vi "multi_channel_DO.vi"(5 "data":u8[][](array[numeric]), 6 "sample num":i32=1000, 7 "sample rate":dbl=1000.0 format="%0.2f", 8 "edge":i32(ring)=10280 items=["上升"=10280, "下降"=10171], 9 "trigger channel":tag, 10 "Trigger Type":enum32{"No Trigger", "Digital Start"}(ring), 11 "channels":tag) -> ()   [LabVIEW 2019]
uses:
  <vilib>/DAQmx/write.llb/DAQmx Write (Digital Wfm 1Chan NSamp).vi
  <vilib>/DAQmx/create/channels.llb/DAQmx Create Channel (DO-Digital Output).vi
  <vilib>/DAQmx/configure/timing.llb/DAQmx Timing (Sample Clock).vi
  <vilib>/DAQmx/configure/trigger.llb/DAQmx Start Trigger (Digital Edge).vi
  <vilib>/Waveform/DWDTOps.llb/DWDT Uncompress Digital.vi
  <vilib>/DAQmx/miscellaneous.llb/DAQmx Fill In Error Info.vi
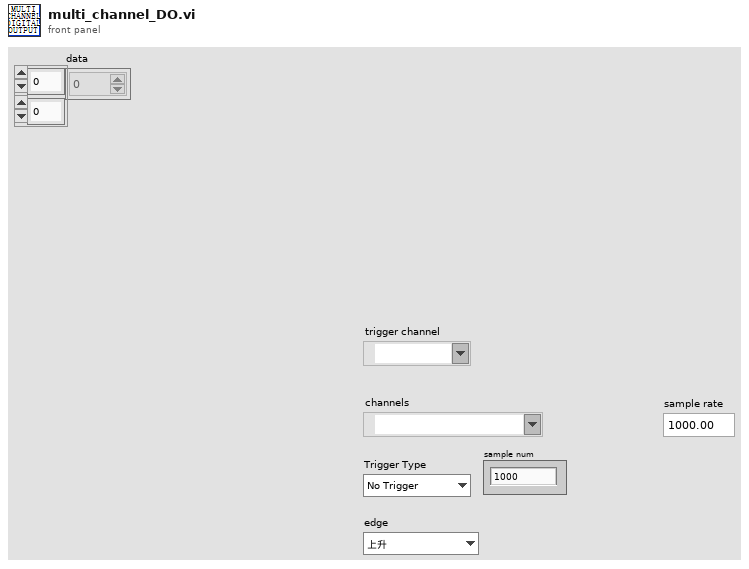
[diagram p1: front panel]
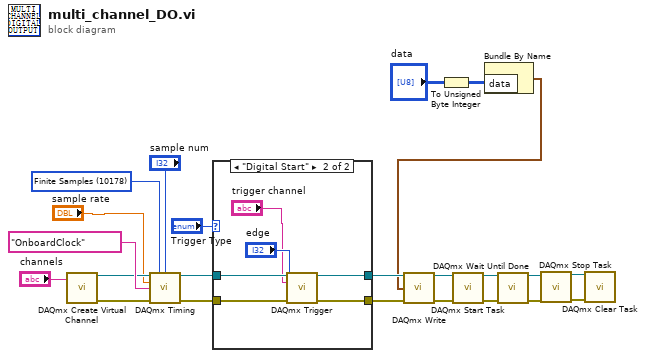
[diagram p0: block diagram]
diagram:
  w5 = 10178 items=["Finite Samples"=10178, "Continuous Samples"=10123, "Hardware Timed Single Point"=12522] ("sample mode")
  n1 = call-poly <vilib>:"DAQmx Create Virtual Channel.vi"("lines"="channels") -> ("task out"=w22:refnum<k21>, "error out"=w21:errorcluster)  [unwired: 13 in]
  n2 = call-poly <vilib>:"DAQmx Timing.vi"("task/channels in"=w22, "sample mode"=w5, "samples per channel"="sample num", "rate"="sample rate", "source"=tag "OnboardClock" ("采样时钟源"), "error in"=w21) -> ("task out"=w17:refnum<k21>, "error out"=w16:errorcluster)  [unwired: 8 in]
  n3 = case shown="\"Digital Start\"" "Trigger Type" {
    tunnel: w17 -> [w25 w31]
    tunnel: w16 -> [w24 w30]
    tunnel: [w25 w28] -> w19
    tunnel: [w24 w27] -> w18
    frame "No Trigger", Default {
    }
    frame "Digital Start" {
      n4 = call-poly <vilib>:"DAQmx Trigger.vi"("task/channels in"=w31, "source"="trigger channel", "edge"="edge", "error in"=w30) -> ("task out"=w28:refnum<k21>, "error out"=w27:errorcluster)  [unwired: 10 in]
    }
  }
  n5 = To Unsigned Byte Integer(number="data") -> (unsigned 8bit integer=w2:u8[][])
  n6 = Bundle By Name("data"=w2) -> (w3:digitaldata)  [unwired: 1 in]
  n7 = call-poly <vilib>:"DAQmx Write.vi"("task/channels in"=w19, "data"=w3, "error in"=w18) -> ("task out"=w11:refnum<k21>, "error out"=w10:errorcluster)  [unwired: 10 in, 1 out]
  n8 = call <vilib>:"DAQmx Start Task.vi"("task/channels in"=w11, "error in"=w10) -> ("task out"=w13:refnum<k21>, "error out"=w12:errorcluster)  [unwired: 12 in]
  n9 = call <vilib>:"DAQmx Wait Until Done.vi"("task/channels in"=w13, "error in"=w12) -> ("task out"=w9:refnum<k21>, "error out"=w8:errorcluster)  [unwired: 12 in]
  n10 = call <vilib>:"DAQmx Stop Task.vi"("task/channels in"=w9, "error in"=w8) -> ("task out"=w7:refnum<k21>, "error out"=w6:errorcluster)  [unwired: 12 in]
  n11 = call <vilib>:"DAQmx Clear Task.vi"("task in"=w7, "error in"=w6) -> ()  [unwired: 13 in, 1 out]
